vi "Remove Unused Terminals On Nodes.vi"(6 "Variant in":variant, 7 "Shift Pressed?":bool, 8 "error in (no error)":errorcluster, 10 "QD Combo Box Ref":refnum<vi>, 11 "QD Launch VI Ref":refnum<vi>) -> (0 "error out":errorcluster, 4 "Variant out":variant)   [LabVIEW 2017, in "Remove Unused Terminals On Nodes.lvlib"]
doc: "Helps people select Bundler nodes, Unbundler nodes and Property nodes to remove unused terminals.\nWorks for:\nBundle By Name (Bundler > NamedBundler)\nBuild Array (Bundler > BuildArray)\nConcatenate Strings (Bundler)\nBundle (Bundler)\nMerge Errors (Bundler)\nUnbundle By Name (Unbundler > NamedUnbundler)\nProperty Node (ObjectFunction > Property)\n\nDefault Shortcut - [Y]"
uses:
  Remove Unused Terminals On Nodes.lvlib
panel:
  in  "Undo Name":string="Quick Drop Remove"
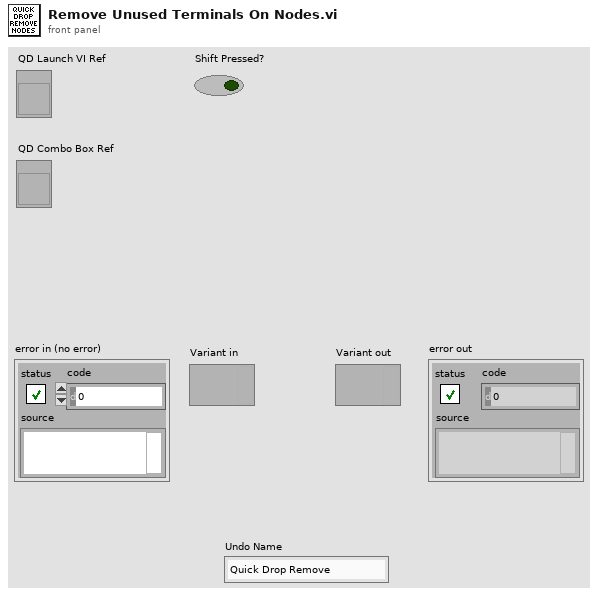
[diagram p1: front panel]
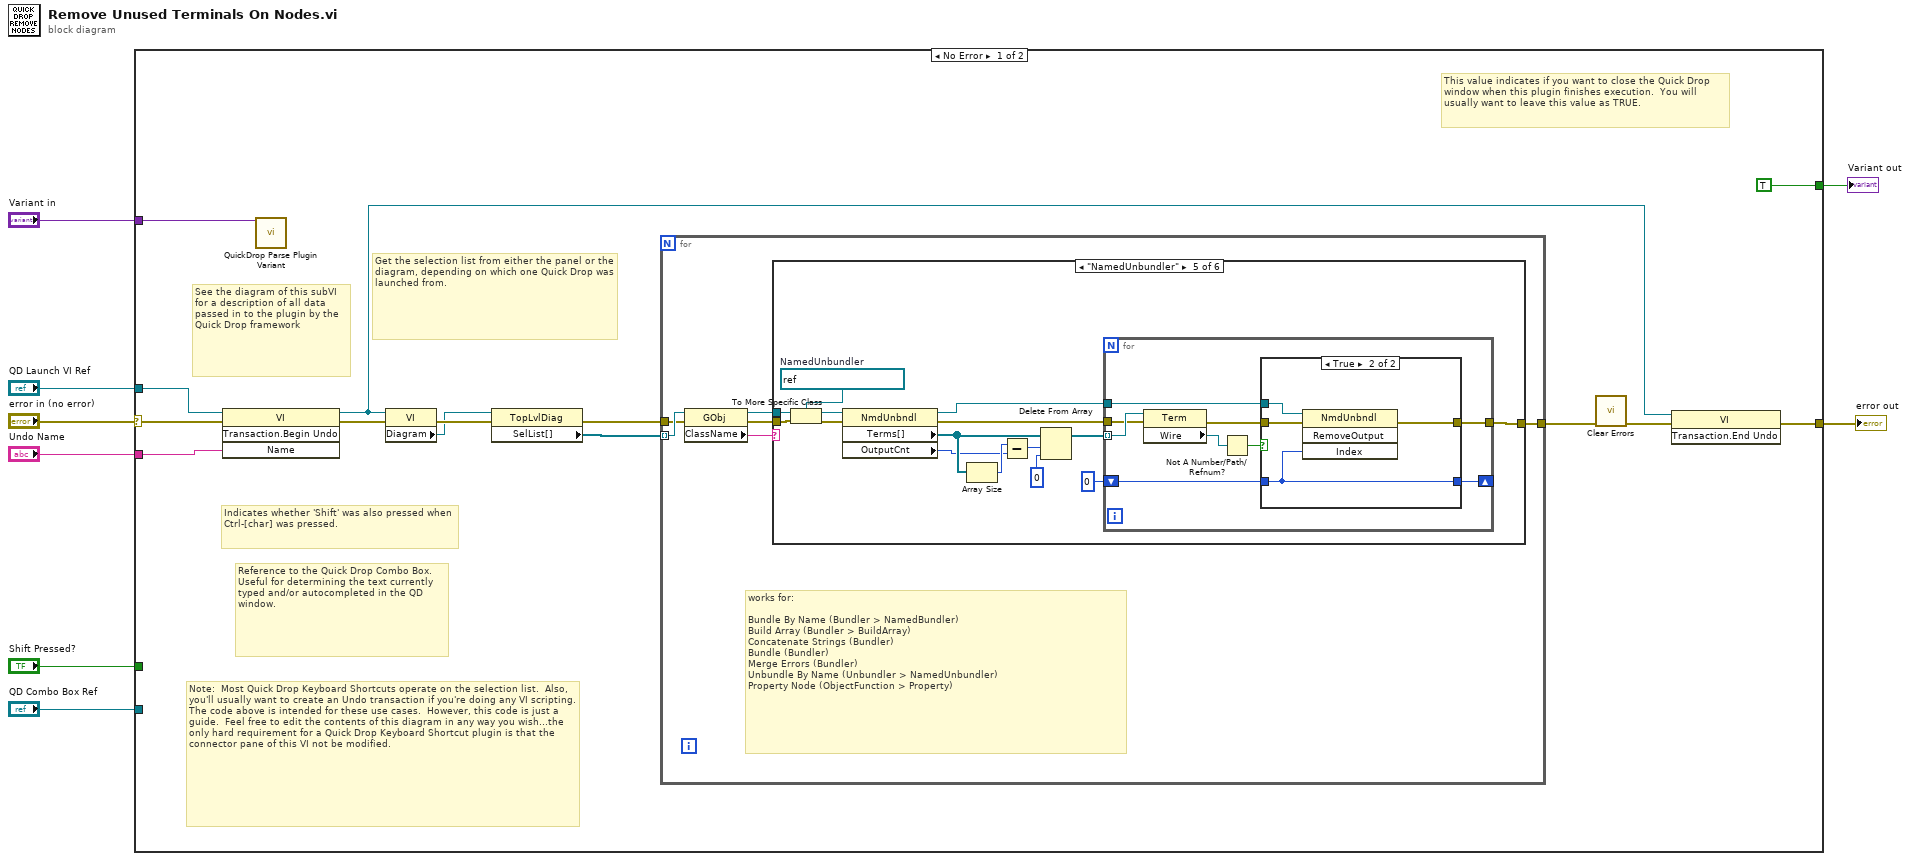
[diagram p0: block diagram]
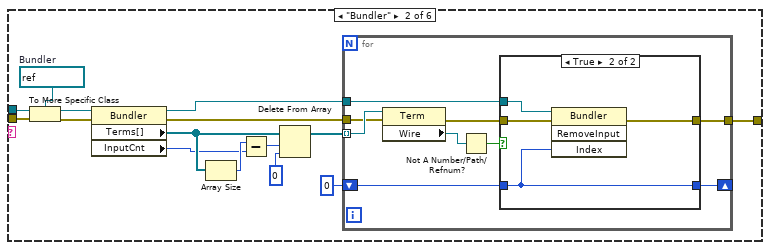
[diagram p3: hidden frame]
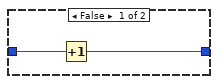
[diagram p4: hidden frame]
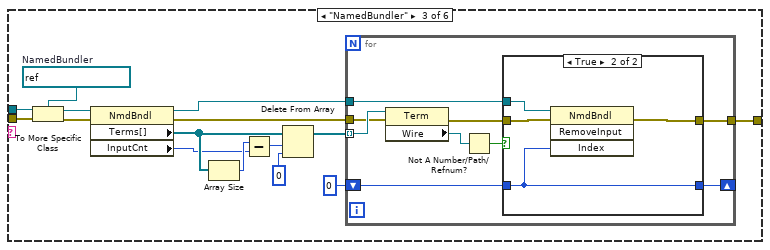
[diagram p5: hidden frame]
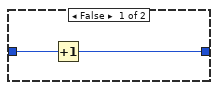
[diagram p6: hidden frame]
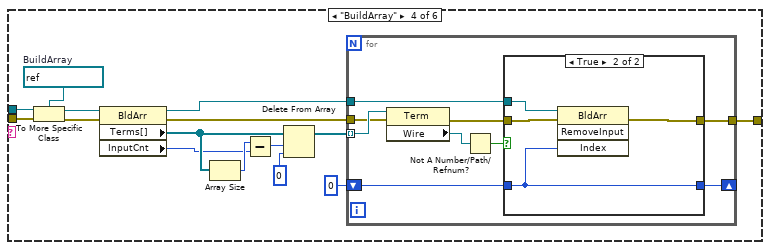
[diagram p7: hidden frame]
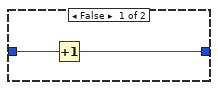
[diagram p8: hidden frame]
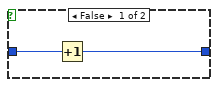
[diagram p9: hidden frame]
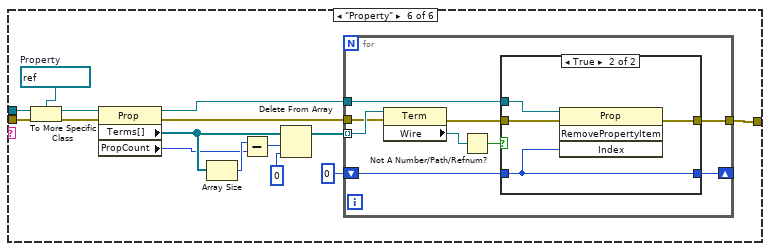
[diagram p10: hidden frame]
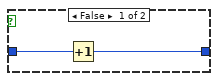
[diagram p11: hidden frame]
diagram:
  n1 = case shown="No Error" "error in (no error)" {
    selector: "error in (no error)" -> [w15 w180]
    tunnel: [w12 w180] -> w7
    tunnel: "QD Launch VI Ref" -> [w16 _]
    tunnel: "Shift Pressed?" -> [_ _]
    tunnel: "QD Combo Box Ref" -> [_ _]
    tunnel: "Undo Name" -> [w14 _]
    tunnel: "Variant in" -> [w17 _]
    tunnel: [TRUE _] -> w1
    frame No Error {
      # "Get the selection list from either the panel or the diagram, depending on which one Quick Drop was launched from."
      # "Note:  Most Quick Drop Keyboard Shortcuts operate on the selection list.  Also, you'll usually want to create an Undo transaction if you're doing any VI scripting.  The code above is intended for these use cases.  However, this code is just a guide.  Feel free to edit the contents of this diagram in any way you wish...the only hard requirement for a Quick Drop Keyboard Shortcut plugin is that the connector pane of this VI not be modified."
      # "This value indicates if you want to close the Quick Drop window when this plugin finishes execution.  You will usually want to leave this value as TRUE."
      # "See the diagram of this subVI for a description of all data passed in to the plugin by the Quick Drop framework"
      # "Reference to the Quick Drop Combo Box.  Useful for determining the text currently typed and/or autocompleted in the QD window."
      # "Indicates whether 'Shift' was also pressed when Ctrl-[char] was pressed."
      n2 = invoke class="VI" method="Transaction.Begin Undo"(reference=w16, error in=w15, "Name"=w14) -> (reference out=w21:refnum<vi>, error out=w22:errorcluster)  [unwired: 1 in, 2 out]
      n3 = call <vilib>:"QuickDrop Parse Plugin Variant.vi"("QDKS Variant in"=w17) -> ()  [unwired: 12 in, 3 out]
      n4 = property class="VI"(reference=w21, error in=w22) -> (error out=w20:errorcluster, "Diagram"=w19:refnum<vi>)  [unwired: 1 out]
      n5 = property class="TopLvlDiag"(reference=w19, error in=w20) -> (error out=w10:errorcluster, "SelList[]"=w18:refnum<vi>[])  [unwired: 1 out]
      n6 = for {
        tunnel: w18 -> [w28] mode=indexing
        tunnel: w10 -> [w24]
        tunnel: [w23] -> w11
        # "works for:\n\nBundle By Name (Bundler > NamedBundler)\nBuild Array (Bundler > BuildArray)\nConcatenate Strings (Bundler)\nBundle (Bundler)\nMerge Errors (Bundler)\nUnbundle By Name (Unbundler > NamedUnbundler)\nProperty Node (ObjectFunction > Property)"
        n7 = property class="GObj"(reference=w28, error in=w24) -> (reference out=w26:refnum<vi>, error out=w25:errorcluster, "ClassName"=w27:string)
        n8 = case shown="\"NamedUnbundler\"" w27 {
          tunnel: w26 -> [_ w31 w62 w91 w125 w152]
          tunnel: w25 -> [w29 w32 w61 w92 w124 w151]
          tunnel: [w29 w30 w60 w90 w122 w150] -> w23
          frame Default {
          }
          frame "Bundler" {
            w36 = refnum<vi> refnum  # Bundler
            n9 = To More Specific Class(target class=w36, reference=w31, error in=w32) -> (specific class reference=w44:refnum<vi>, error out=w34:errorcluster)
            n10 = property class="Bundler"(reference=w44, error in=w34) -> (reference out=w37:refnum<vi>, error out=w33:errorcluster, "Terms[]"=w38:refnum<vi>[], "InputCnt"=w35:i32)
            n11 = Array Size(array=w38) -> (size(s)=w41:i32)
            n12 = Subtract(x=w41, y=w35) -> (x-y=w42:i32)
            n13 = Delete From Array(array=w38, length=w42, index=0) -> (array with subset deleted=w43:refnum<vi>[])  [unwired: 1 out]
            n14 = for {
              tunnel: w43 -> [w53] mode=indexing
              shift-right: [w49] -> _
              shift-left: 0 -> [w50]
              tunnel: w37 -> [w48]
              tunnel: [w47] -> w30
              tunnel: w33 -> [w45]
              n15 = property class="Term"(reference=w53, error in=w45) -> (error out=w46:errorcluster, "Wire"=w52:refnum<vi>)  [unwired: 1 out]
              n16 = Not A Number/Path/Refnum?(number/path/refnum=w52) -> (NaN/Path/Refnum?=w51:bool)
              n17 = case shown="True" w51 {
                tunnel: w50 -> [w55 w58]
                tunnel: [w54 w58] -> w49
                tunnel: w48 -> [_ w59]
                tunnel: [_ w57] -> w47
                tunnel: w46 -> [_ w56]
                frame False {
                  n18 = Increment(x=w55) -> (x+1=w54:i32)
                }
                frame True {
                  n19 = invoke class="Bundler" method="RemoveInput"(reference=w59, error in=w56, "Index"=w58) -> (error out=w57:errorcluster)  [unwired: 1 in, 3 out]
                }
              }
            }
          }
          frame "NamedBundler" {
            w66 = refnum<vi> refnum  # NamedBundler
            n20 = To More Specific Class(target class=w66, reference=w62, error in=w61) -> (specific class reference=w74:refnum<vi>, error out=w64:errorcluster)
            n21 = property class="NmdBndl"(reference=w74, error in=w64) -> (reference out=w67:refnum<vi>, error out=w63:errorcluster, "Terms[]"=w68:refnum<vi>[], "InputCnt"=w65:i32)
            n22 = Array Size(array=w68) -> (size(s)=w71:i32)
            n23 = Subtract(x=w71, y=w65) -> (x-y=w72:i32)
            n24 = Delete From Array(array=w68, length=w72, index=0) -> (array with subset deleted=w73:refnum<vi>[])  [unwired: 1 out]
            n25 = for {
              tunnel: w73 -> [w83] mode=indexing
              shift-right: [w79] -> _
              shift-left: 0 -> [w80]
              tunnel: w67 -> [w78]
              tunnel: [w77] -> w60
              tunnel: w63 -> [w75]
              n26 = property class="Term"(reference=w83, error in=w75) -> (error out=w76:errorcluster, "Wire"=w82:refnum<vi>)  [unwired: 1 out]
              n27 = Not A Number/Path/Refnum?(number/path/refnum=w82) -> (NaN/Path/Refnum?=w81:bool)
              n28 = case shown="True" w81 {
                tunnel: w80 -> [w85 w88]
                tunnel: [w84 w88] -> w79
                tunnel: w78 -> [_ w89]
                tunnel: [_ w87] -> w77
                tunnel: w76 -> [_ w86]
                frame False {
                  n29 = Increment(x=w85) -> (x+1=w84:i32)
                }
                frame True {
                  n30 = invoke class="NmdBndl" method="RemoveInput"(reference=w89, error in=w86, "Index"=w88) -> (error out=w87:errorcluster)  [unwired: 1 in, 3 out]
                }
              }
            }
          }
          frame "BuildArray" {
            w96 = refnum<vi> refnum  # BuildArray
            n31 = To More Specific Class(target class=w96, reference=w91, error in=w92) -> (specific class reference=w104:refnum<vi>, error out=w94:errorcluster)
            n32 = property class="BldArr"(reference=w104, error in=w94) -> (reference out=w97:refnum<vi>, error out=w93:errorcluster, "Terms[]"=w98:refnum<vi>[], "InputCnt"=w95:i32)
            n33 = Array Size(array=w98) -> (size(s)=w101:i32)
            n34 = Subtract(x=w101, y=w95) -> (x-y=w102:i32)
            n35 = Delete From Array(array=w98, length=w102, index=0) -> (array with subset deleted=w103:refnum<vi>[])  [unwired: 1 out]
            n36 = for {
              tunnel: w103 -> [w113] mode=indexing
              shift-right: [w109] -> _
              shift-left: 0 -> [w110]
              tunnel: w97 -> [w108]
              tunnel: [w107] -> w90
              tunnel: w93 -> [w105]
              n37 = property class="Term"(reference=w113, error in=w105) -> (error out=w106:errorcluster, "Wire"=w112:refnum<vi>)  [unwired: 1 out]
              n38 = Not A Number/Path/Refnum?(number/path/refnum=w112) -> (NaN/Path/Refnum?=w111:bool)
              n39 = case shown="True" w111 {
                tunnel: w110 -> [w115 w118]
                tunnel: [w114 w118] -> w109
                tunnel: w108 -> [_ w119]
                tunnel: [_ w117] -> w107
                tunnel: w106 -> [_ w116]
                frame False {
                  n40 = Increment(x=w115) -> (x+1=w114:i32)
                }
                frame True {
                  n41 = invoke class="BldArr" method="RemoveInput"(reference=w119, error in=w116, "Index"=w118) -> (error out=w117:errorcluster)  [unwired: 1 in, 3 out]
                }
              }
            }
          }
          frame "NamedUnbundler" {
            w126 = refnum<vi> refnum  # NamedUnbundler
            n42 = To More Specific Class(target class=w126, reference=w125, error in=w124) -> (specific class reference=w134:refnum<vi>, error out=w121:errorcluster)
            n43 = property class="NmdUnbndl"(reference=w134, error in=w121) -> (reference out=w127:refnum<vi>, error out=w120:errorcluster, "Terms[]"=w128:refnum<vi>[], "OutputCnt"=w123:i32)
            n44 = Array Size(array=w128) -> (size(s)=w131:i32)
            n45 = Subtract(x=w131, y=w123) -> (x-y=w132:i32)
            n46 = Delete From Array(array=w128, length=w132, index=0) -> (array with subset deleted=w133:refnum<vi>[])  [unwired: 1 out]
            n47 = for {
              tunnel: w133 -> [w143] mode=indexing
              shift-right: [w139] -> _
              shift-left: 0 -> [w140]
              tunnel: w127 -> [w138]
              tunnel: [w137] -> w122
              tunnel: w120 -> [w135]
              n48 = property class="Term"(reference=w143, error in=w135) -> (error out=w136:errorcluster, "Wire"=w142:refnum<vi>)  [unwired: 1 out]
              n49 = Not A Number/Path/Refnum?(number/path/refnum=w142) -> (NaN/Path/Refnum?=w141:bool)
              n50 = case shown="True" w141 {
                tunnel: w140 -> [w145 w148]
                tunnel: [w144 w148] -> w139
                tunnel: w138 -> [_ w149]
                tunnel: [_ w147] -> w137
                tunnel: w136 -> [_ w146]
                frame False {
                  n51 = Increment(x=w145) -> (x+1=w144:i32)
                }
                frame True {
                  n52 = invoke class="NmdUnbndl" method="RemoveOutput"(reference=w149, error in=w146, "Index"=w148) -> (error out=w147:errorcluster)  [unwired: 1 in, 3 out]
                }
              }
            }
          }
          frame "Property" {
            w156 = refnum<vi> refnum  # Property
            n53 = To More Specific Class(target class=w156, reference=w152, error in=w151) -> (specific class reference=w164:refnum<vi>, error out=w154:errorcluster)
            n54 = property class="Prop"(reference=w164, error in=w154) -> (reference out=w157:refnum<vi>, error out=w153:errorcluster, "Terms[]"=w158:refnum<vi>[], "PropCount"=w155:i32)
            n55 = Array Size(array=w158) -> (size(s)=w161:i32)
            n56 = Subtract(x=w161, y=w155) -> (x-y=w162:i32)
            n57 = Delete From Array(array=w158, length=w162, index=0) -> (array with subset deleted=w163:refnum<vi>[])  [unwired: 1 out]
            n58 = for {
              tunnel: w163 -> [w173] mode=indexing
              shift-right: [w169] -> _
              shift-left: 0 -> [w170]
              tunnel: w157 -> [w168]
              tunnel: [w167] -> w150
              tunnel: w153 -> [w165]
              n59 = property class="Term"(reference=w173, error in=w165) -> (error out=w166:errorcluster, "Wire"=w172:refnum<vi>)  [unwired: 1 out]
              n60 = Not A Number/Path/Refnum?(number/path/refnum=w172) -> (NaN/Path/Refnum?=w171:bool)
              n61 = case shown="True" w171 {
                tunnel: w170 -> [w175 w178]
                tunnel: [w174 w178] -> w169
                tunnel: w168 -> [_ w179]
                tunnel: [_ w177] -> w167
                tunnel: w166 -> [_ w176]
                frame False {
                  n62 = Increment(x=w175) -> (x+1=w174:i32)
                }
                frame True {
                  n63 = invoke class="Prop" method="RemovePropertyItem"(reference=w179, error in=w176, "Index"=w178) -> (error out=w177:errorcluster)  [unwired: 1 in, 3 out]
                }
              }
            }
          }
        }
      }
      n64 = call <vilib>:"Clear Errors.vi"("error in (no error)"=w11) -> ("error out"=w9:errorcluster)  [unwired: 5 in, 1 out]
      n65 = invoke class="VI" method="Transaction.End Undo"(reference=w21, error in=w9) -> (error out=w12:errorcluster)  [unwired: 1 in, 2 out]
    }
    frame Error {
    }
  }
  "error out" <- w7
  "Variant out" <- w1
